vi "scale_host_test.vi"() -> ()   [LabVIEW 2025]
panel:
  out "16bit integer":i16
  in  "factor":u16
  in  "val":fxp<+/-,18,1>
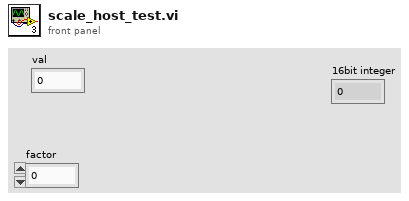
[diagram p1: front panel]
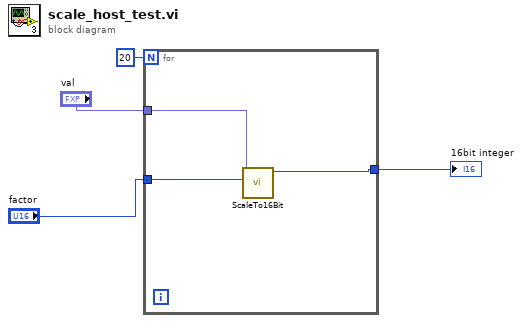
[diagram p0: block diagram]
diagram:
  n1 = for {
    N: 20 -> [_]
    tunnel: "val" -> [w7]
    tunnel: "factor" -> [w6]
    tunnel: [w5] -> w2
    n2 = call "ScaleTo16Bit.vi"("factor"=w6, "val"=w7) -> ("16bit integer"=w5:i16)  [unwired: 8 in, 1 out]
  }
  "16bit integer" <- w2
